vi "Generic Camera Get Image Info.vi"(0 "Image Ref":T1, 11 "Error In":errorcluster) -> (4 "Image Ref Dup":T1, 8 "Camera Image Info":T2, 15 "Error Out":errorcluster)   [LabVIEW 2025]
uses:
  <vilib>/vision/Image Controls.llb/IMAQ Image.ctl
  Camera Controls/Camera IMAQ Key Info.ctl
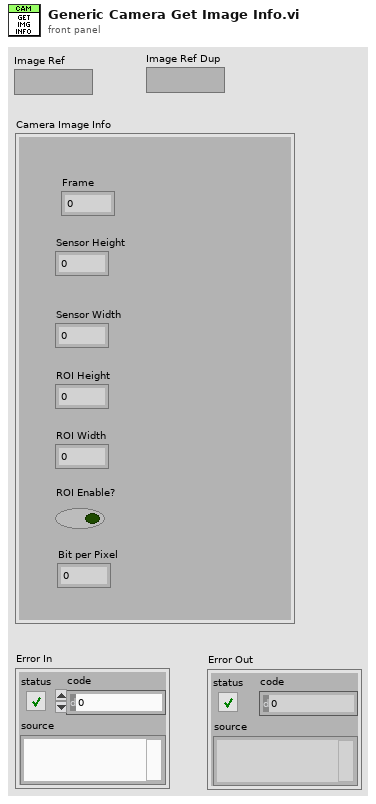
[diagram p1: front panel]
types:
  T1 = typedef "IMAQ Image.ctl" = refnum<image>
  T2 = typedef "Camera IMAQ Key Info.ctl" = cluster{"Frame":u32, "Sensor Height":i32, "Sensor Width":i32, "ROI Height":i32, "ROI Width":i32, "ROI Enable?":bool, "Bit per Pixel":u8}
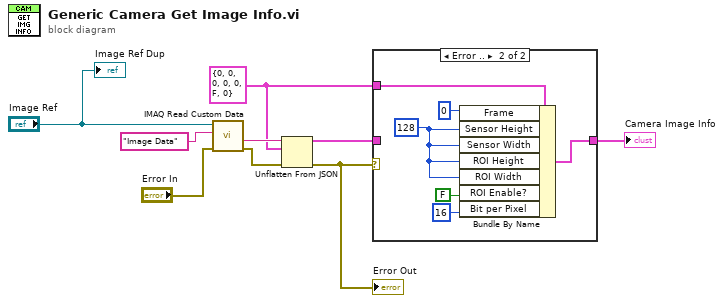
[diagram p0: block diagram]
diagram:
  w3 = T2 {"Frame"=0, "Sensor Height"=0, "Sensor Width"=0, "ROI Height"=0, "ROI Width"=0, "ROI Enable?"=FALSE, "Bit per Pixel"=0} ("Camera IMAQ Key Info")
  n1 = call "IMAQ Read Custom Data"("error in (no error)"="Error In", "Key"="Image Data", "Image"="Image Ref") -> ("error out"=w6:errorcluster, "Custom Data Out"=w7:string)  [unwired: 6 in, 1 out]
  n2 = Unflatten From JSON(JSON string=w7, type and defaults=w3, error in (no error)=w6) -> (value=w5:T2, error out=w1:errorcluster)  [unwired: 4 in]
  "Error Out" <- w1
  n3 = case shown="Error .." w1 {
    tunnel: w5 -> [w10 _]
    tunnel: [w10 w11] -> w4
    tunnel: w3 -> [_ w16]
    frame No Error {
    }
    frame Error {
      w14 = 128 ("Sensor Height")
      n4 = Bundle By Name(cluster=w16, "Frame"=u32 0, "Sensor Height"=w14, "Sensor Width"=w14, "ROI Height"=w14, "ROI Width"=w14, "ROI Enable?"=FALSE, "Bit per Pixel"=u8 16) -> (w11:T2)
    }
  }
  "Camera Image Info" <- w4
  "Image Ref Dup" <- "Image Ref"
